vi "Health and fitness analyzer.vi"() -> ()   [LabVIEW 2020]
panel:
  in  "COM Port":refnum<visa-resource-name>
  out "Heart rate":dbl(graph)
  out "Temperature":dbl(graph)
  out "Temperature":dbl(slide) scale=0.0..50.0
  in  "Patient's record":string[][](table)
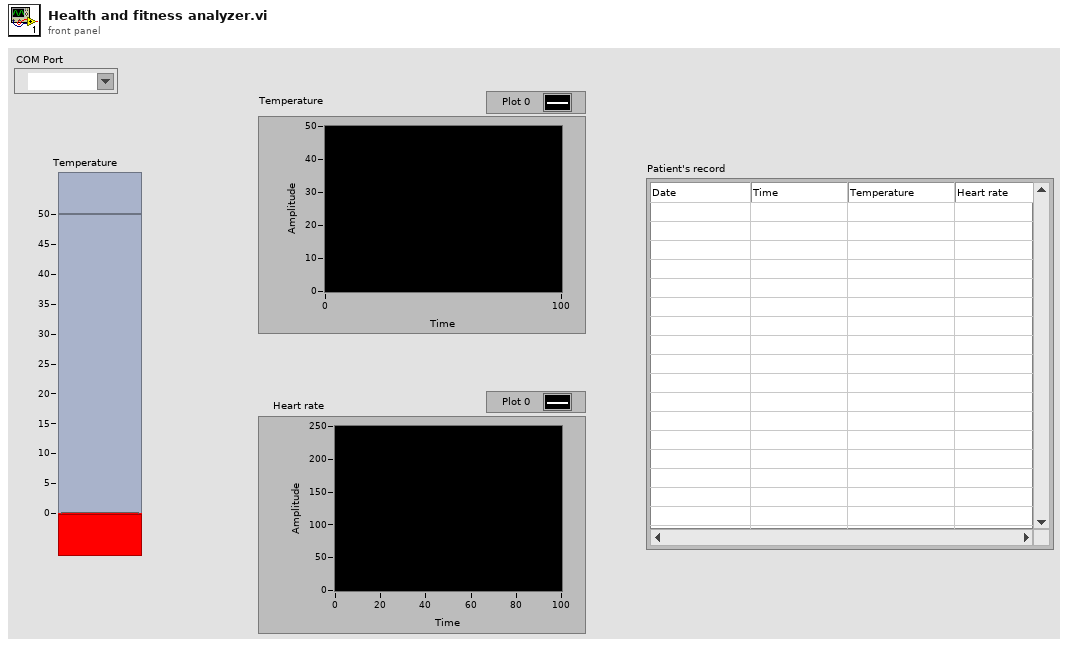
[diagram p1: front panel]
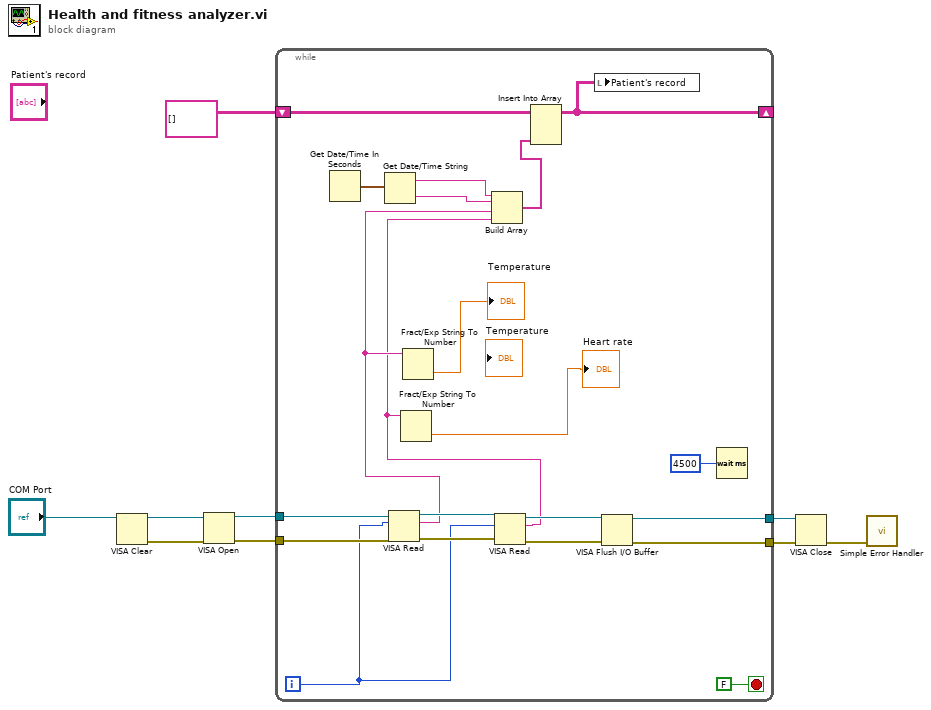
[diagram p0: block diagram]
diagram:
  n1 = VISA Clear(VISA resource name="COM Port") -> (VISA resource name out=w9:refnum<visa-resource-name>, error out=w8:errorcluster)  [unwired: 1 in]
  n2 = VISA Open(error in (no error)=w8, VISA resource name=w9) -> (VISA resource name=w7:refnum<visa-resource-name>, error out=w6:errorcluster)  [unwired: 3 in]
  n3 = while {
    tunnel: w7 -> [w28]
    tunnel: w6 -> [w27]
    tunnel: [w24] -> w5
    tunnel: [w23] -> w4
    shift-right: [w11] -> _
    shift-left: string[][] [] -> [w12]
    i -> [w22]
    stop <- FALSE stop-if-true
    n4 = Get Date/Time In Seconds() -> (seconds since 1Jan1904=w18:timestamp)
    n5 = Get Date/Time String(seconds (now)=w18) -> (date string=w17:string, time string=w16:string)  [unwired: 2 in]
    n6 = VISA Read(VISA resource name=w28, byte count=w22, error in (no error)=w27) -> (VISA resource name out=w30:refnum<visa-resource-name>, read buffer=w15:string, error out=w29:errorcluster)  [unwired: 1 out]
    n7 = Fract/Exp String To Number(string=w15) -> (number=→"Temperature":dbl)  [unwired: 3 in, 1 out]
    n8 = VISA Read(VISA resource name=w30, byte count=w22, error in (no error)=w29) -> (VISA resource name out=w26:refnum<visa-resource-name>, read buffer=w14:string, error out=w25:errorcluster)  [unwired: 1 out]
    n9 = Fract/Exp String To Number(string=w14) -> (number=→"Heart rate":dbl)  [unwired: 3 in, 1 out]
    n10 = Build Array(w17, w16, w15, w14) -> (w13:string[])
    n11 = Insert Into Array(array=w12, new element=w13) -> (w11:string[][])  [unwired: 2 in]
    n12 = local write "Patient's record"(w11) -> ()
    n13 = VISA Flush I/O Buffer(VISA resource name=w26, error in (no error)=w25) -> (VISA resource name out=w24:refnum<visa-resource-name>, error out=w23:errorcluster)  [unwired: 1 in]
    n14 = Wait (ms)(milliseconds to wait=u32 4500) -> ()  [unwired: 1 out]
  }
  n15 = VISA Close(VISA resource name=w5, error in (no error)=w4) -> (error out=w3:errorcluster)
  n16 = call <vilib>:"Simple Error Handler.vi"("error in (no error)"=w3) -> ()  [unwired: 4 in, 5 out]
